vi "startTcpServerB.vi"(8 "error in (no error)":errorcluster, 11 "TcpServer.lvclass":refnum<class "TcpServer.lvclass">) -> (0 "error out":errorcluster, 2 "TcpServer out":refnum<class "TcpServer.lvclass">, 3 "UserEvents":T1)   [LabVIEW 2018]
doc: "Start the TCP server B."
uses:
  src/TcpServer/TcpServer.lvclass
  src/TcpServerBase/typedef/connStatusCluster.ctl
  src/TcpServerBase/TcpServerBase.lvclass
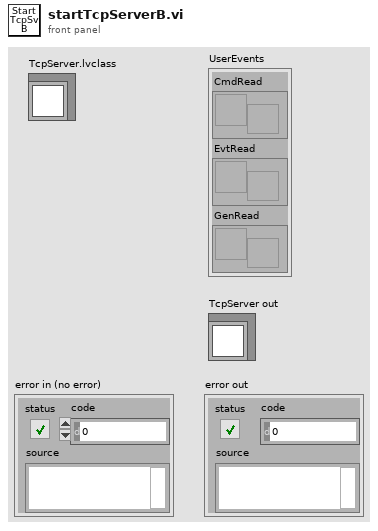
[diagram p1: front panel]
types:
  T1 = cluster{"CmdRead":refnum<user-event>, "EvtRead":refnum<user-event>, "GenRead":refnum<user-event>}
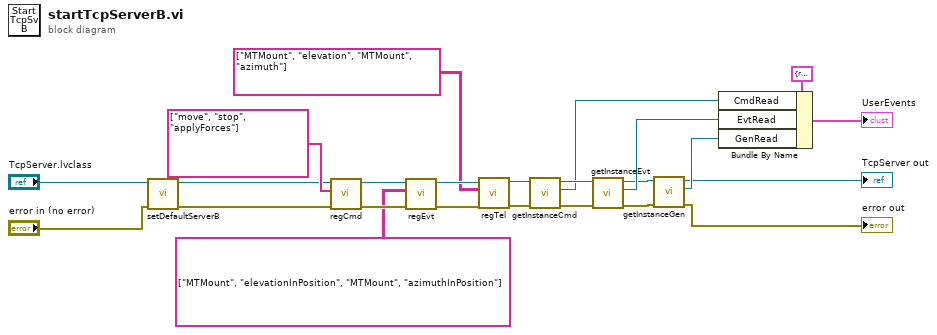
[diagram p0: block diagram]
diagram:
  n1 = call "setDefaultServerB.vi"("error in (no error)"="error in (no error)", "TcpServer.lvclass"="TcpServer.lvclass") -> ("error out"=w3:errorcluster, "tcpServer out"=w2:refnum<class "TcpServer.lvclass">)  [unwired: 8 in]
  n2 = call "regCmd.vi"("error in (no error)"=w3, "cmdReg"=string[] ["move", "stop", "applyForces"], "tcpServer in"=w2) -> ("error out"=w20:errorcluster, "tcpServer out"=w21:refnum<class "TcpServer.lvclass">)  [unwired: 7 in]
  n3 = call "regEvt.vi"("error in (no error)"=w20, "evtReg"=string[][] [["MTMount", "elevationInPosition"], ["MTMount", "azimuthInPosition"]], "tcpServer in"=w21) -> ("error out"=w17:errorcluster, "tcpServer out"=w18:refnum<class "TcpServer.lvclass">)  [unwired: 7 in]
  n4 = call "regTel.vi"("error in (no error)"=w17, "telReg"=string[][] [["MTMount", "elevation"], ["MTMount", "azimuth"]] ("regTel"), "tcpServer in"=w18) -> ("error out"=w14:errorcluster, "tcpServer out"=w15:refnum<class "TcpServer.lvclass">)  [unwired: 7 in]
  n5 = call "getInstanceCmd.vi"("error in (no error)"=w14, "tcpServer in"=w15) -> ("error out"=w12:errorcluster, "CmdRead"=w11:refnum<user-event>, "tcpServer out"=w13:refnum<class "TcpServer.lvclass">)  [unwired: 7 in]
  n6 = call "getInstanceEvt.vi"("error in (no error)"=w12, "tcpServer in"=w13) -> ("error out"=w8:errorcluster, "EvtRead"=w10:refnum<user-event>, "tcpServer out"=w9:refnum<class "TcpServer.lvclass">)  [unwired: 7 in]
  n7 = call "getInstanceGen.vi"("error in (no error)"=w8, "tcpServer in"=w9) -> ("error out"=→"error out":errorcluster, "GenRead"=w7:refnum<user-event>, "tcpServer out"=→"TcpServer out":refnum<class "TcpServer.lvclass">)  [unwired: 7 in]
  n8 = Bundle By Name(cluster=T1 {"CmdRead"=refnum, "EvtRead"=refnum, "GenRead"=refnum}, "CmdRead"=w11, "EvtRead"=w10, "GenRead"=w7) -> (→"UserEvents":T1)
